vi "2-6-3.vi"() -> ()   [LabVIEW 2022 SP3]
panel:
  out "布尔":bool
  out "数值":dbl
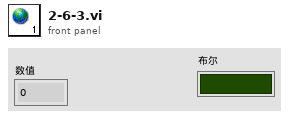
[diagram p1: front panel]
diagram:
